vi "Untitled 1.vi"() -> ()   [LabVIEW 2019]
panel:
  in  "stop":bool
  in  "Temperature(F)":dbl(slide) scale=0.0..200.0
  out "Thermometer(C)":dbl(slide) scale=0.0..100.0
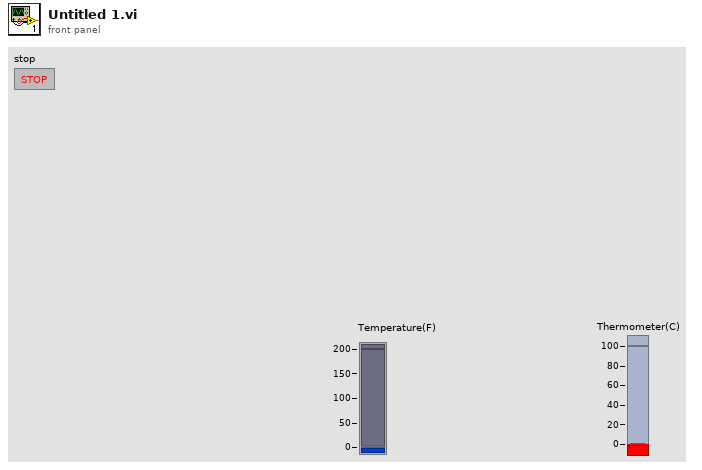
[diagram p1: front panel]
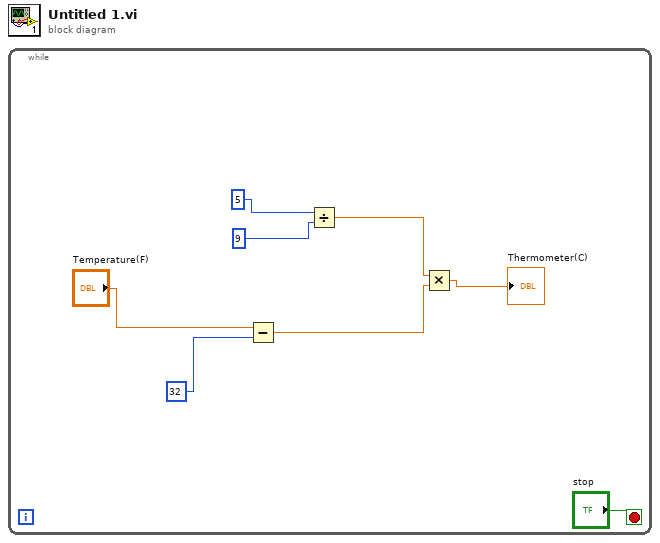
[diagram p0: block diagram]
diagram:
  n1 = while {
    stop <- "stop" stop-if-true
    n2 = Subtract(x="Temperature(F)", y=32) -> (x-y=w3:dbl)
    n3 = Divide(x=5, y=9) -> (x/y=w4:dbl)
    n4 = Multiply(x=w4, y=w3) -> (x*y=→"Thermometer(C)":dbl)
  }
